vi "FTW-CodeGen-Image.vi"(0 "State In":T1, 5 "XRef":refnum<vi>) -> (4 "Image":picture)   [LabVIEW 2015, in "FTW-JSON-Fetch.xnode"]
uses:
  FTW-JSON-Fetch.xnode
  FTW-CodeGen-State.ctl
  FTW-CodeGen-XNodeCommonState.ctl
panel:
  # "Inputs"
  # "Outputs"
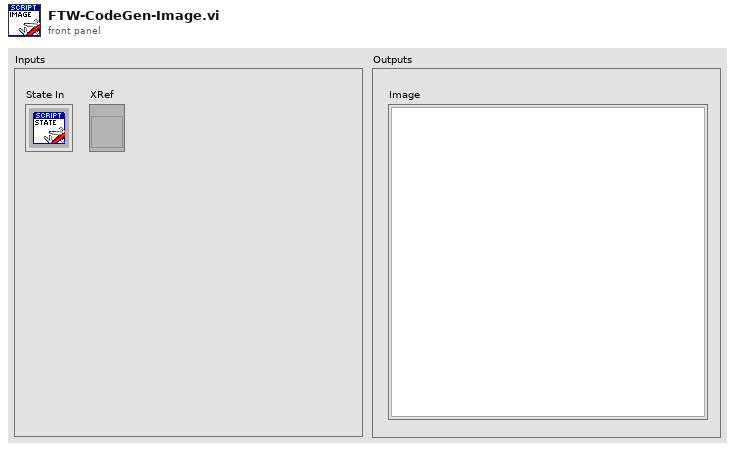
[diagram p1: front panel]
types:
  T1 = typedef "FTW-JSON-Fetch.xnode/FTW-CodeGen-State.ctl" = cluster{"Cache":T2, "JSONObjectAdaptiveTermIndex":i32, "ElementAdaptiveTermIndex":i32, "PathTermIndex":i32}
  T2 = typedef "FTW-CodeGen-XNodeCommonState.ctl" = cluster{"Terms":cluster{"Name":string, "Id":string, "Type":variant, "Bounds":cluster{"Left":i32, "Top":i32, "Right":i32, "Bottom":i32}, "Input?":bool, "Required?":bool, "Recommended?":bool, "Adaptive?":bool, "Hidden?":bool, "Direction":enum32{"Auto", "Up", "Down", "Left", "Right", "Center"}, "Break Wire?":bool, "English Name":string}[], "AdaptiveTerms":string[], "AdaptedTypes":variant[], "ForceCodeRegeneration?":bool, "LastGeneration":timestamp, "Errors":string[]}
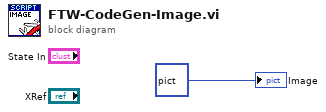
[diagram p0: block diagram]
diagram:
  "Image" <- picture bytes[3230] ("new picture")
